vi "xmlFull.vi"(0 "TDD?":bool, 1 "single spec":dbl[](array[numeric]), 2 "Points":dbl[](array[numeric]), 4 "file path (dialog if empty)":path caption="文件路径 （空时为对话框）", 5 "TDD spec":string, 6 "limit type":enum16{"上限", "下限"}(ring), 7 "SN":string, 8 "ABS?":bool, 9 "数组":string[](array[string])=["Port1-Port2: TD-RD", "Port1-Port2: RD-TD"], 10 "second result":string) -> (3 "OutPutXml":string)   [LabVIEW 2011]
uses:
  <vilib>/Utility/file.llb/Read From Spreadsheet File (string).vi
panel:
  out "所用时间":dbl
  out "all rows":string[][](array[string]) caption="所有行"
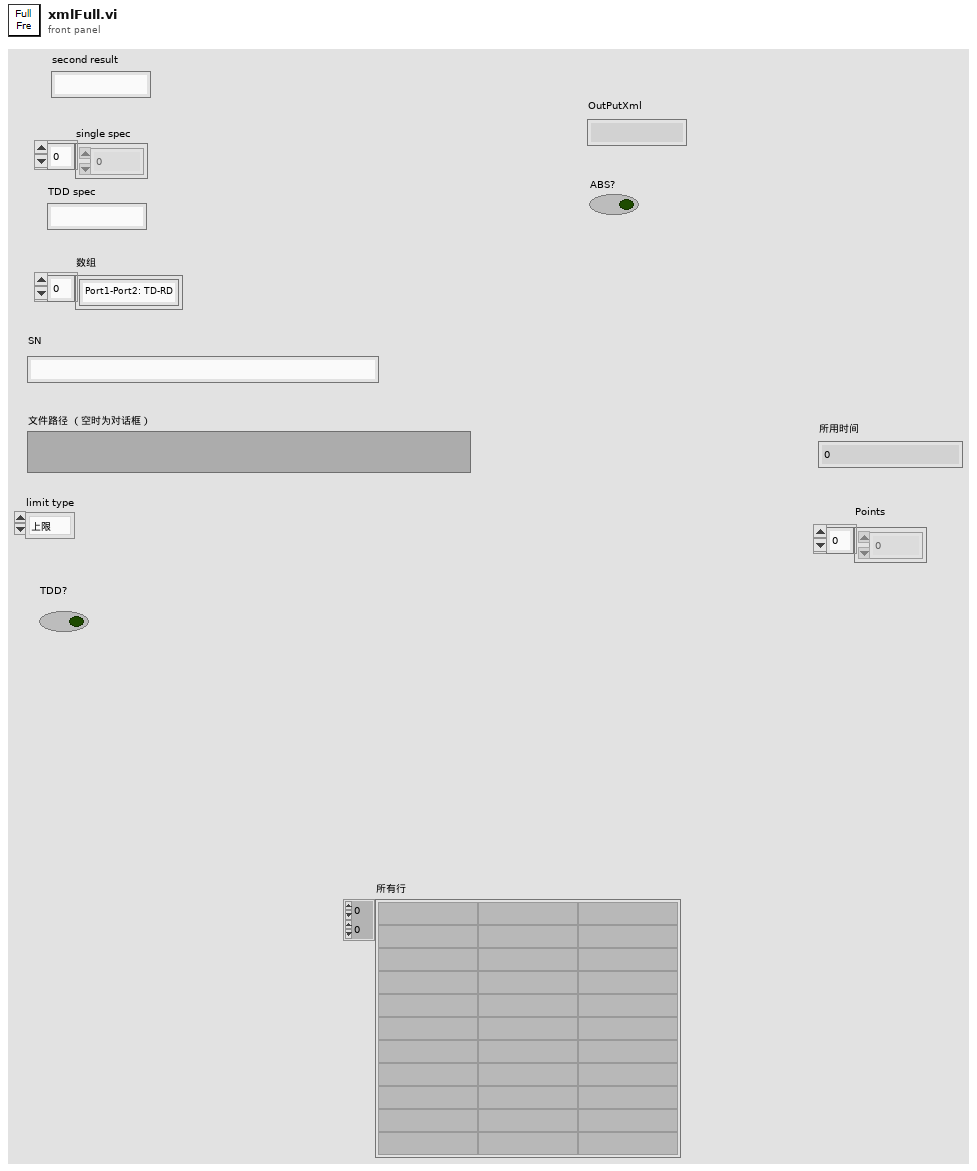
[diagram p1: front panel]
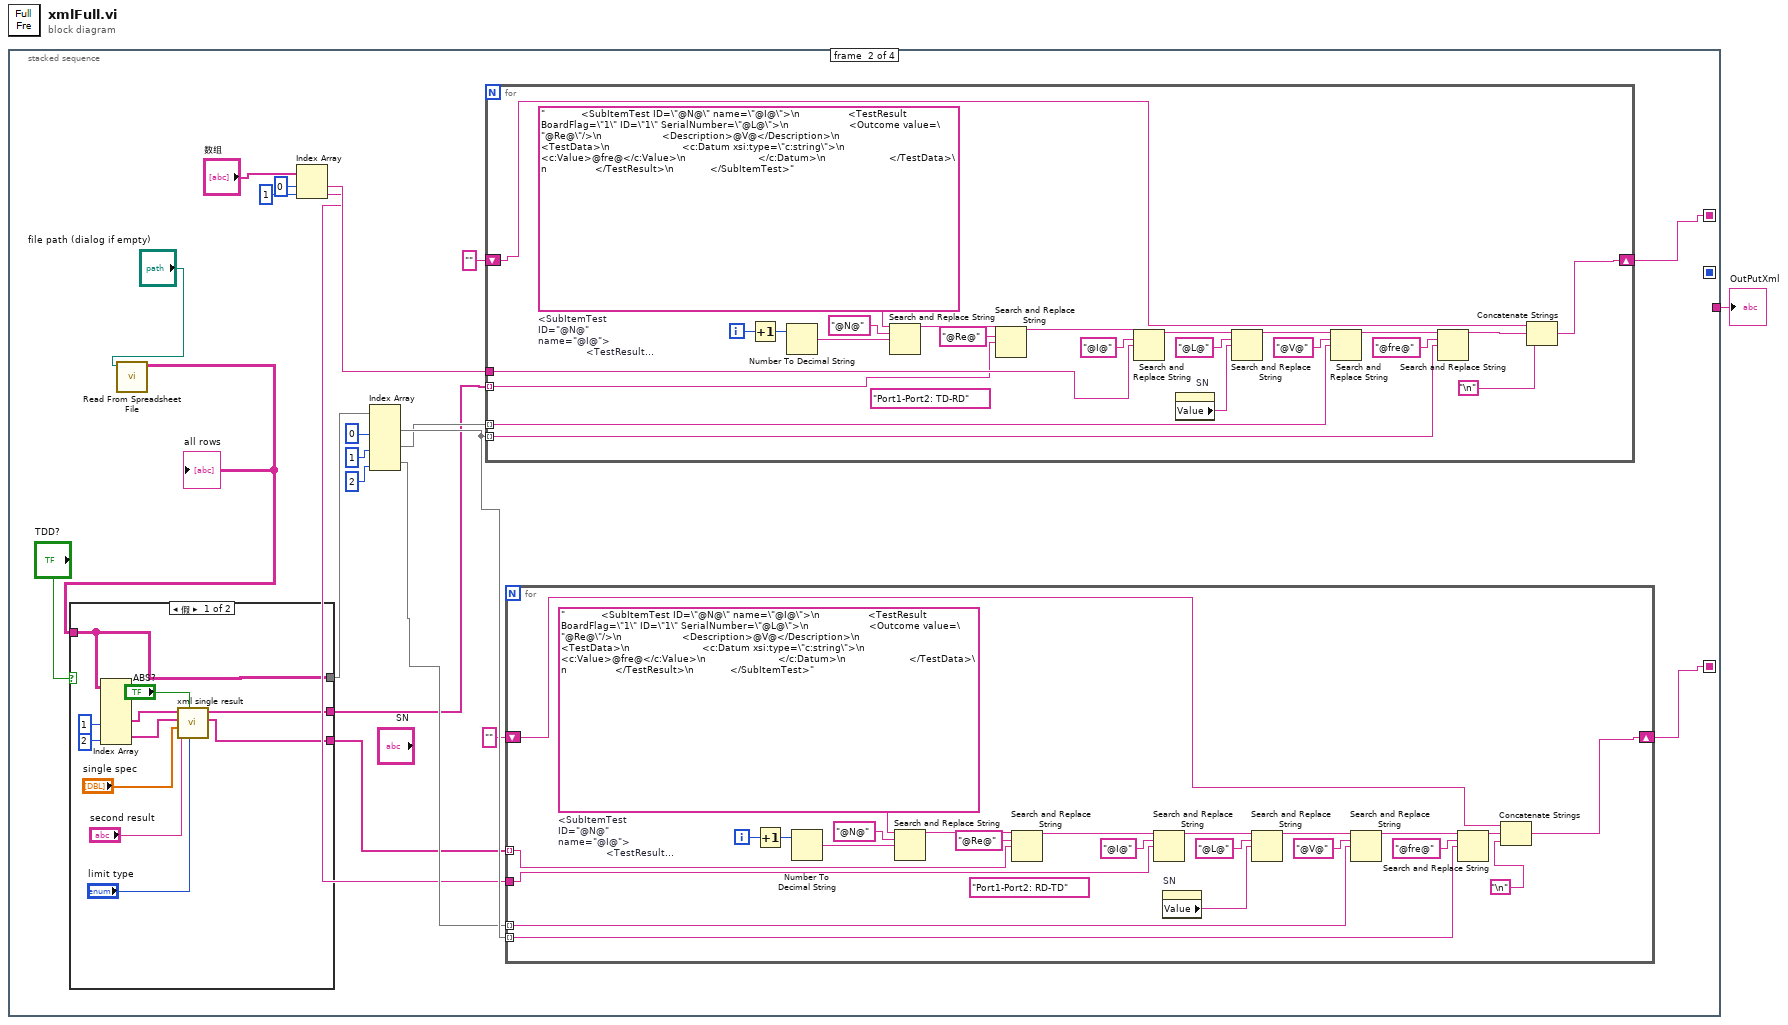
[diagram p0: block diagram]
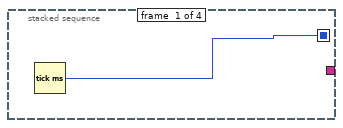
[diagram p2: hidden frame]
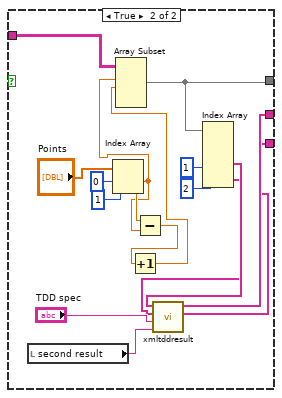
[diagram p3: hidden frame]
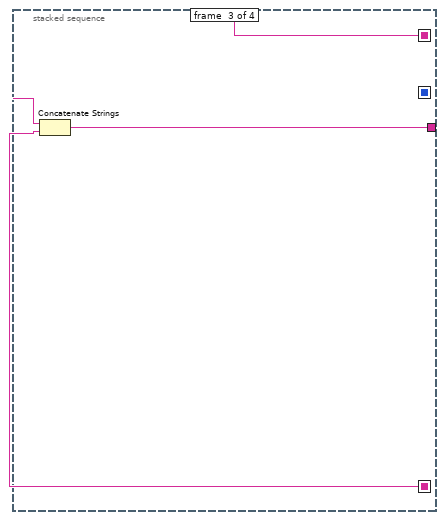
[diagram p4: hidden frame]
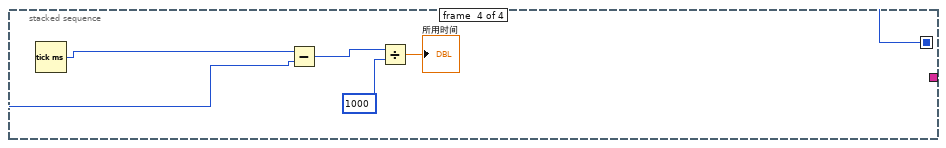
[diagram p5: hidden frame]
diagram:
  n1 = stacked-sequence {
    seq-local: [w2 _ _ _] -> [_ _ _ w106]
    seq-local: [_ w17 _ _] -> [_ _ w102 _]
    seq-local: [_ w16 _ _] -> [_ _ w101 _]
    tunnel: [_ _ w100 _] -> w1
    frame #0 {
      n2 = Tick Count (ms)() -> (millisecond timer value=w2:u32)
    }
    frame #1 {
      n3 = call-poly <vilib>:"Read From Spreadsheet File.vi"("file path (dialog if empty)"="file path (dialog if empty)") -> ("all rows"=w7:string[][])  [unwired: 6 in, 4 out]
      "all rows" <- w7
      n4 = case shown="假" "TDD?" {
        tunnel: w7 -> [w34 w51]
        tunnel: [w34 w41] -> w6
        tunnel: [w27 w36] -> w4
        tunnel: [w26 w35] -> w3
        frame False {
          n5 = Index Array(array=w34, index (col) #2=1 ("禁用的索引 (列)"), index (col) #3=2 ("索引 (列)")) -> (element #2=w31:string[], element #3=w30:string[])  [unwired: 4 in, 1 out]
          n6 = call "xml single result.vi"("limit type"="limit type", "ABS?"="ABS?", "second result"="second result", "single spec"="single spec", "TX data"=w30, "RX data"=w31) -> ("TX array"=w26:string[], "RX array"=w27:string[])  [unwired: 4 in]
        }
        frame True {
          n7 = local read "second result"() -> (w43:string)
          n8 = Index Array(array="Points", index #1=0 ("索引"), index #2=1 ("索引")) -> (element #1=w46:dbl, element #2=w47:dbl)
          n9 = Subtract(x=w47, y=w46) -> (x-y=w45:dbl)
          n10 = Increment(x=w45) -> (x+1=w44:dbl)
          n11 = Array Subset(array=w51, index (row)=w46, length (row)=w44) -> (w41:string[][])  [unwired: 2 in]
          n12 = Index Array(array=w41, index (col) #2=1 ("禁用的索引 (列)"), index (col) #3=2 ("索引 (列)")) -> (element #2=w38:string[], element #3=w37:string[])  [unwired: 4 in, 1 out]
          n13 = call "xmltddresult.vi"("second result"=w43, "TDD spec"="TDD spec", "TX data"=w37, "RX data"=w38) -> ("TX array"=w35:string[], "RX array"=w36:string[])  [unwired: 6 in]
        }
      }
      n14 = Index Array(array="数组", index #1=0 ("索引"), index #2=1 ("索引")) -> (element #1=w10:string, element #2=w9:string)
      n15 = Index Array(array=w6, index (col) #1=0 ("禁用的索引 (列)"), index (col) #2=1 ("索引 (列)"), index (col) #3=2 ("索引 (列)")) -> (element #1=w19:string[], element #2=w5:string[], element #3=w18:string[])  [unwired: 3 in]
      n16 = for {
        tunnel: w5 -> [w88] mode=indexing
        tunnel: w19 -> [w84] mode=indexing
        shift-right: [w82] -> w17
        shift-left: "" -> [w81]
        tunnel: w10 -> [w80]
        tunnel: w4 -> [w76] mode=indexing
        i -> [w90]
        (unwired) "Port1-Port2: TD-RD" ("替换字符串(\"\")")
        w99 = "            <SubItemTest ID=\"@N@\" name=\"@I@\">\n                <TestResult BoardFlag=\"1\" ID=\"1\" SerialNumber=\"@L@\">\n                    <Outcome value=\"@Re@\"/>\n                    <Description>@V@</Description>\n                    <TestData>\n                        <c:Datum xsi:type=\"c:string\">\n                            <c:Value>@fre@</c:Value>\n                        </c:Datum>\n                     </TestData>\n                </TestResult>\n            </SubItemTest>"  # <SubItemTest ID="@N@" name="@I@">                 <TestResult BoardFlag="1" ID="1" SerialNumber="@L@">                     <Outcome value="@Re@"/>                     <Description>@V@</Description>                     <TestData>                         <c:Datum xsi:type="c:string">                             <c:Value>@fre@</c:Value>                         </c:Datum>                      </TestData>                 </TestResult>             </SubItemTest>
        n17 = Increment(x=w90) -> (x+1=w92:i32)
        n18 = Number To Decimal String(number=w92) -> (decimal integer string=w97:string)  [unwired: 1 in]
        n19 = Search and Replace String(input string=w99, search string="@N@" ("搜索字符串"), replace string=w97) -> (result string=w79:string)  [unwired: 5 in, 3 out]
        n20 = Search and Replace String(input string=w79, search string="@Re@" ("搜索字符串"), replace string=w76) -> (result string=w77:string)  [unwired: 5 in, 3 out]
        n21 = Search and Replace String(input string=w77, search string="@I@" ("搜索字符串"), replace string=w80) -> (result string=w95:string)  [unwired: 5 in, 3 out]
        n22 = property on="SN" class="Str"() -> ("Value"=w89:string)  [unwired: 2 in, 2 out]
        n23 = Search and Replace String(input string=w95, search string="@L@" ("搜索字符串"), replace string=w89) -> (result string=w91:string)  [unwired: 5 in, 3 out]
        n24 = Search and Replace String(input string=w91, search string="@V@" ("搜索字符串"), replace string=w88) -> (result string=w87:string)  [unwired: 5 in, 3 out]
        n25 = Search and Replace String(input string=w87, search string="@fre@" ("搜索字符串"), replace string=w84) -> (result string=w86:string)  [unwired: 5 in, 3 out]
        n26 = Concatenate Strings(w81, w86, "\n") -> (w82:string)
      }
      n27 = for {
        tunnel: w18 -> [w65] mode=indexing
        tunnel: w19 -> [w61] mode=indexing
        shift-right: [w58] -> w16
        shift-left: "" -> [w57]
        tunnel: w9 -> [w56]
        tunnel: w3 -> [w52] mode=indexing
        i -> [w66]
        (unwired) "Port1-Port2: RD-TD" ("替换字符串(\"\")")
        w75 = "            <SubItemTest ID=\"@N@\" name=\"@I@\">\n                <TestResult BoardFlag=\"1\" ID=\"1\" SerialNumber=\"@L@\">\n                    <Outcome value=\"@Re@\"/>\n                    <Description>@V@</Description>\n                    <TestData>\n                        <c:Datum xsi:type=\"c:string\">\n                            <c:Value>@fre@</c:Value>\n                        </c:Datum>\n                     </TestData>\n                </TestResult>\n            </SubItemTest>"  # <SubItemTest ID="@N@" name="@I@">                 <TestResult BoardFlag="1" ID="1" SerialNumber="@L@">                     <Outcome value="@Re@"/>                     <Description>@V@</Description>                     <TestData>                         <c:Datum xsi:type="c:string">                             <c:Value>@fre@</c:Value>                         </c:Datum>                      </TestData>                 </TestResult>             </SubItemTest>
        n28 = Increment(x=w66) -> (x+1=w68:i32)
        n29 = Number To Decimal String(number=w68) -> (decimal integer string=w73:string)  [unwired: 1 in]
        n30 = Search and Replace String(input string=w75, search string="@N@" ("搜索字符串"), replace string=w73) -> (result string=w55:string)  [unwired: 5 in, 3 out]
        n31 = Search and Replace String(input string=w55, search string="@Re@" ("搜索字符串"), replace string=w52) -> (result string=w54:string)  [unwired: 5 in, 3 out]
        n32 = Search and Replace String(input string=w54, search string="@I@" ("搜索字符串"), replace string=w56) -> (result string=w71:string)  [unwired: 5 in, 3 out]
        n33 = property on="SN" class="Str"() -> ("Value"=w60:string)  [unwired: 2 in, 2 out]
        n34 = Search and Replace String(input string=w71, search string="@L@" ("搜索字符串"), replace string=w60) -> (result string=w67:string)  [unwired: 5 in, 3 out]
        n35 = Search and Replace String(input string=w67, search string="@V@" ("搜索字符串"), replace string=w65) -> (result string=w64:string)  [unwired: 5 in, 3 out]
        n36 = Search and Replace String(input string=w64, search string="@fre@" ("搜索字符串"), replace string=w61) -> (result string=w63:string)  [unwired: 5 in, 3 out]
        n37 = Concatenate Strings(w57, w63, "\n") -> (w58:string)
      }
    }
    frame #2 {
      n38 = Concatenate Strings(w102, w101) -> (w100:string)
    }
    frame #3 {
      n39 = Tick Count (ms)() -> (millisecond timer value=w107:u32)
      n40 = Subtract(x=w107, y=w106) -> (x-y=w105:u32)
      n41 = Divide(x=w105, y=u32 1000) -> (x/y=→"所用时间":dbl)
    }
  }
  "OutPutXml" <- w1
